vi "SetAttributeViInt32.vi"(7 "AttributeValue":i32 format="%.0g", 8 "error in (no error)":errorcluster {"code" format="%.0x"}, 9 "AttributeID":u32(ring)=1150006 items=["ALARM_MODE"=1150006, "ALARM_SLOPE"=1150007, "FORMAT_TIME_MODE"=1150026, "ROUTE_MONITOR_VIEW"=1150068, "SCAN_CHANNEL_ADVANCE_SOURCE"=1150028, "SCAN_READING_THRESHOLD"=1150031, "SCAN_SINGLE_CHANNEL_SAMPLE_COUNT_PRE_TRIGGER"=1150063, "SCAN_SINGLE_CHANNEL_SAMPLE_COUNT"=1150062, "SCAN_SWEEP_COUNT"=1150008, "SCAN_TRIGGER_OUTPUT_SLOPE"=1150067, "SCAN_TRIGGER_SLOPE"=1150061, "SCAN_TRIGGER_SOURCE"=1150009, "STATUS_ALARM_ENABLE_REGISTER"=1150040, "STATUS_OPERATION_ENABLE_REGISTER"=1150044, "STATUS_QUESTIONABLE_ENABLE_REGISTER"=1150045, "STATUS_SERVICE_REQUEST_ENABLE_REGISTER"=1150047, "STATUS_STANDARD_EVENT_ENABLE_REGISTER"=1150046, "SYSTEM_AUTOCALIBRATION_MONTHLY_INTERVAL_DAY"=1150049, "SYSTEM_AUTOCALIBRATION_OCCURENCE_INTERVAL"=1150048, "SYSTEM_AUTOCALIBRATION_WEEKLY_INTERVAL_DAY"=1150050, "SYSTEM_IO_TIMEOUT"=1150002, "SYSTEM_TRACING_LEVEL"=1150043, "USB_MEMORY_COLUMN_HEADER"=1150054, "USB_MEMORY_COLUMN_SEPARATOR"=1150035, "USB_MEMORY_ROW_LIMIT_COUNT"=1150055], 11 "instrument handle":refnum<k15>) -> (0 "error out":errorcluster {"code" format="%.0x"}, 3 "instrument handle out":refnum<k15>)   [LabVIEW 2020, in "Keysight DAQ970.lvlib"]
doc: "Sets an Int32 attribute from the instrument driver.\nThe following Attributes are supported:\n\nALARM_MODE\n\nALARM_SLOPE\n\nFORMAT_TIME_MODE\n\nROUTE_MONITOR_VIEW \n\nSCAN_CHANNEL_ADVANCE_SOURCE\n\nSCAN_READING_THRESHOLD\n\nSCAN_SINGLE_CHANNEL_SAMPLE_COUNT_PRE_TRIGGER\n\nSCAN_SINGLE_CHANNEL_SAMPLE_COUNT\n\nSCAN_SWEEP_COUNT\n\nSCAN_TRIGGER_OUTPUT_SLOPE\n\nSCAN_TRIGGER_SLOPE\n\nSCAN_TRIGGER_SOURCE\n\nSTATUS_ALARM_ENABLE_REGISTER\n\nSTATUS_OPERATION_ENABLE_REGISTER\n\nSTATUS_QUESTIONABLE_ENABLE_REGISTER\n\nSTATUS_SERVICE_REQUEST_ENABLE_REGISTER\n\nSTATUS_STANDARD_EVENT_ENABLE_REGISTER\n\nSYSTEM_AUTOCALIBRATION_MONTHLY_INTERVAL_DAY\n\nSYSTEM_AUTOCALIBRATION_OCCURENCE_INTERVAL\n\nSYSTEM_AUTOCALIBRATION_WEEKLY_INTERVAL_DAY\n\nSYSTEM_IO_TIMEOUT\n\nSYSTEM_TRACING_LEVEL\n\nUSB_MEMORY_COLUMN_HEADER\n\nUSB_MEMORY_COLUMN_SEPARATOR\n\nUSB_MEMORY_ROW_LIMIT_COUNT"
uses:
  Keysight DAQ970.lvlib
  KtDAQ970.dll
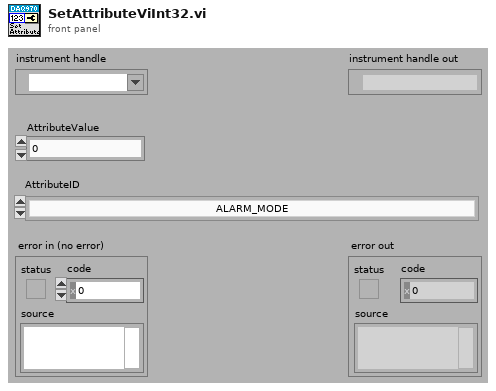
[diagram p1: front panel]
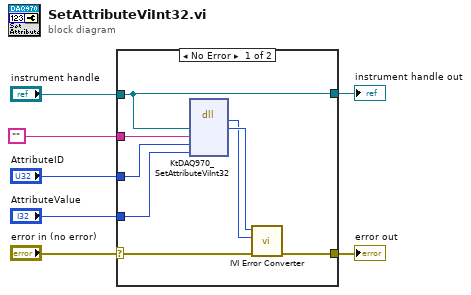
[diagram p0: block diagram]
diagram:
  n1 = case shown="No Error" "error in (no error)" {
    selector: "error in (no error)" -> [w13 w17]
    tunnel: [w12 w17] -> w7
    tunnel: "instrument handle" -> [w8 w16]
    tunnel: "" -> [w11 _]
    tunnel: "AttributeID" -> [w10 _]
    tunnel: "AttributeValue" -> [w9 _]
    tunnel: [w8 w16] -> w2
    frame No Error {
      n2 = dll-call lib="KtDAQ970**.dll" fn="KtDAQ970_SetAttributeViInt32"("Vi"=w8, "RepCapIdentifier"=w11, "AttributeID"=w10, "AttributeValue"=w9) -> ("return type"=w14:i32, "Vi"=w15:u32)  [unwired: 6 in, 2 out]
      n3 = call "IVI Error Converter.vi"("error in (no error)"=w13, "IVI error code (0)"=w14, "instrument handle"=w15) -> ("error out"=w12:errorcluster)  [unwired: 7 in, 1 out]
    }
    frame Error {
    }
  }
  "error out" <- w7
  "instrument handle out" <- w2
